vi "GUI_laptop v10.vi"() -> ()   [LabVIEW 2019]
uses:
  <vilib>/Math Plots/3D Math Plots/3D Scatter/3D Scatter XCtrl/3D Scatter.xctl
  <vilib>/Platform/TimedLoop/XDataNode/timing_clust.ctl
  <vilib>/Platform/TimedLoop/XDataNode/nitl_modes.ctl
  <vilib>/Platform/TimedLoop/XDataNode/wakeup.ctl
  <vilib>/Analysis/_algsub.llb/Real Vector Norm.vi
  <vilib>/Instr/_visa.llb/VISA Configure Serial Port (Instr).vi
  <vilib>/Utility/file.llb/Write Delimited Spreadsheet (DBL).vi
  <vilib>/Math Plots/3D Math Plots/3D Scatter/3D Scatter Datatype/Public/Plot Helper (Vector).vi
  <vilib>/platform/TimedLoop/XDataNode/XDataNode.xnode
  <vilib>/Platform/TimedLoop/XDataNode/XDNodeRunTimeDep.lvlib
  <vilib>/Analysis/NI_AALPro.lvlib
  <vilib>/Math Plots/3D Math Plots/3D Scatter/3D Scatter Datatype/3D Scatter Datatype.lvclass
panel:
  out "send values":dbl[](array[numeric])
  out "Robot Feedback (xyz)":dbl[](array[numeric])
  in  "UDP Send":bool
  in  "UDP Recv":bool
  in  "L5 bound":dbl=1000.0
  in  "L4 bound (deg)":dbl=1000.0
  in  "L3 bound (mm)":dbl=1000.0
  in  "L2 bound (deg)":dbl=1000.0
  in  "L1 bound (deg)":dbl=1000.0
  in  "Joystick Type":dbl(ring) items=["Rigid Joystick", "Free Joystick"]
  out "Finished Late? [i-1]":bool
  in  "Epsilon":dbl=0.2
  out "3D Scatter":refnum<class "3D Plot Datatype.lvclass">[](xcontrol)
  out "Random Point":dbl[](array[numeric])
  out "Virtual Cursor":dbl[](array[numeric])
  out "Iteration Duration":i64
  in  "Num of Points":i32=10
  in  "z bound":dbl=2.0
  in  "y bound":dbl=5.0
  in  "x bound":dbl=5.0
  in  "Stop":bool
  in  "Round Decimals":dbl=2.0 format="%#_15g"
  in  "Save  Data":bool
  in  "Save Path":path
  in  "x speed":dbl=0.5
  in  "z speed":dbl=0.5
  in  "y speed":dbl=0.5
  out "error out":errorcluster
  in  "baud rate":u32=115200
  in  "VISA resource name":refnum<visa-resource-name>
  # "TODO: fix the bounds; currently bounds are arbitrary"
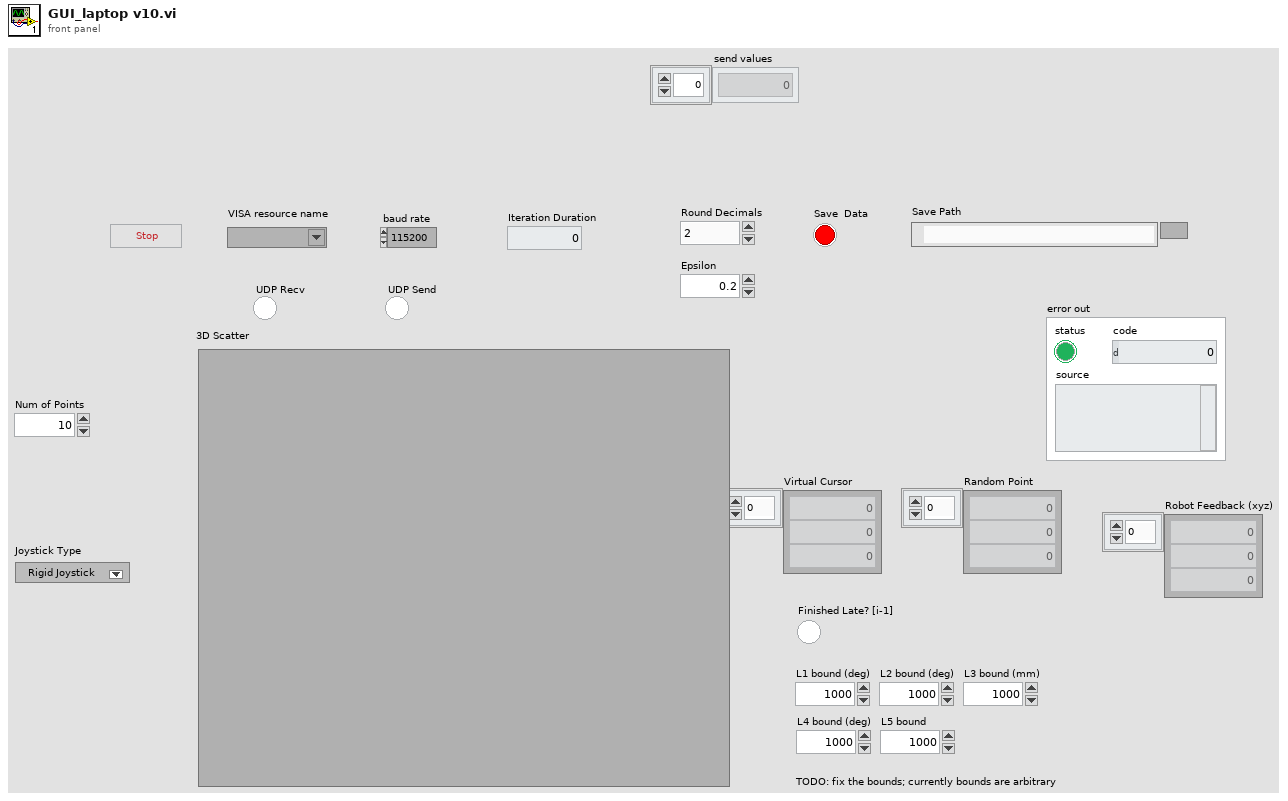
[diagram p1: front panel]
types:
  T1 = typedef "XDNodeRunTimeDep.lvlib/timing_clust.ctl" = cluster{"Expected End [f-1]":u64, "Actual End [f-1]":u64, "Finished Late? [f-1]":bool, "Expected End [i-1]":u64, "Actual End [i-1]":u64, "Finished Late? [i-1]":bool, "Expected Start [i]":u64, "Actual Start [i]":u64, "Expected Start [f]":u64, "Actual Start [f]":u64, "Source Name":string, "Structure Name":string, "Period":i64, "Deadline":i64, "Offset":i64, "Start":i64, "Priority":i32, "Timeout":i32, "Mode":T2, "Wakeup Reason":T3, "Error":errorcluster, "Source Type":string, "Secondary Source Type":string, "Global End Time":u64, "Global Start Time":u64, "Frame Duration":u64, "Iteration Duration":u64, "Assigned CPU":i32, "I/O Scan Engine Mode":u32}
  T2 = typedef "XDNodeRunTimeDep.lvlib/nitl_modes.ctl" = enum32{"No Change", "Process missed periods, maintain original phase", "Discard missed periods, maintain original phase", "Process missed periods, ignore original phase", "Discard missed periods, ignore original phase"}
  T3 = typedef "XDNodeRunTimeDep.lvlib/wakeup.ctl" = enum32{"Normal", "Aborted", "Asynchronous wakeup", "Timing source error", "Timed loop error", "Timeout"}
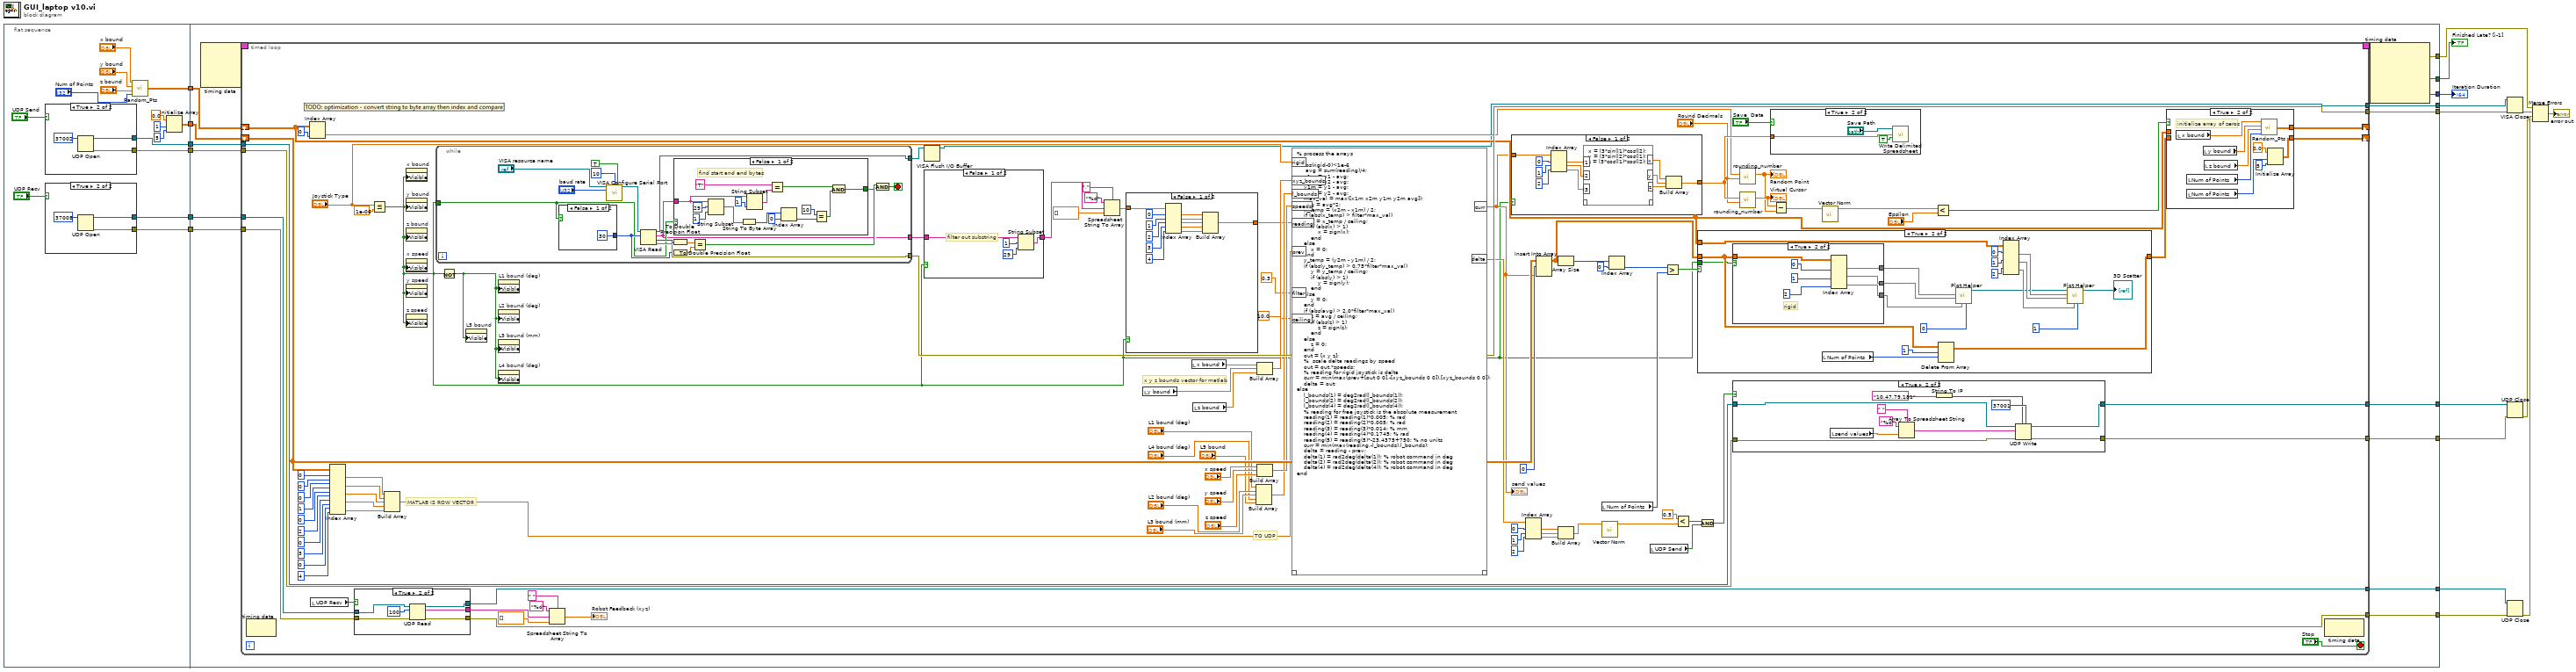
[diagram p0: block diagram]
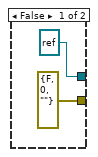
[diagram p2: hidden frame]
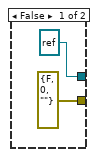
[diagram p3: hidden frame]
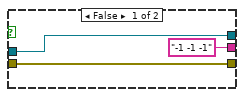
[diagram p5: hidden frame]
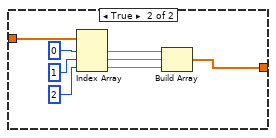
[diagram p9: hidden frame]
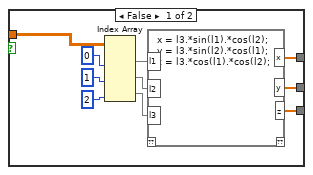
[diagram p12: hidden frame]
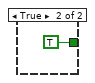
[diagram p13: hidden frame]
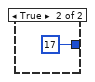
[diagram p14: hidden frame]
diagram:
  n1 = flat-sequence {
    tunnel: [w26] -> w15
    tunnel: [w30] -> w14
    tunnel: [w25] -> w13
    tunnel: [w24] -> w12
    tunnel: [w21] -> w11
    tunnel: [w20] -> w10
    tunnel: [w59] -> w19
    tunnel: [w58] -> w18
    tunnel: [w56] -> w9
    tunnel: [w54] -> w17
    tunnel: [w53] -> w16
    tunnel: w15 -> [w57]
    tunnel: w14 -> [w55]
    tunnel: w13 -> [w52]
    tunnel: w12 -> [w51]
    tunnel: w11 -> [w50]
    tunnel: w10 -> [w49]
    tunnel: [w48] -> w3
    tunnel: [w47] -> w8
    tunnel: [w46] -> w2
    tunnel: [w45] -> w1
    frame #0 {
      n2 = case shown="True" "UDP Send" {
        tunnel: [refnum<k16> refnum ("port") w38] -> w25
        tunnel: [errorcluster {"status"=FALSE, "code"=0, "source"=""} ("error out") w37] -> w20
        frame False {
        }
        frame True {
          n3 = UDP Open(11:u16 37002 ("port")) -> (port=w38:refnum<k16>, 0:w37:errorcluster)  [unwired: 4 in, 1 out]
        }
      }
      n4 = case shown="True" "UDP Recv" {
        tunnel: [refnum<k16> refnum ("port") w43] -> w24
        tunnel: [errorcluster {"status"=FALSE, "code"=0, "source"=""} ("error out") w42] -> w21
        frame False {
        }
        frame True {
          n5 = UDP Open(11:u16 37008 ("port")) -> (port=w43:refnum<k16>, 0:w42:errorcluster)  [unwired: 4 in, 1 out]
        }
      }
      n6 = call "Random_Pts.vi"("Num of Points"="Num of Points", "z bound"="z bound", "y bound"="y bound", "x bound"="x bound") -> ("appended array"=w30:dbl[][])
      n7 = Initialize Array(0.0 ("element"), 1 ("dimension size"), 5 ("dimension size")) -> (w26:dbl[][])
    }
    frame #1 {
      n8 = node-c288() -> (w61:T1)  [unwired: 4 in]
      n9 = timed-loop {
        tunnel: [w94] -> w59
        tunnel: [w158] -> w58
        shift-right: [w157] -> _
        shift-left: w57 -> [w156]
        timing: w61 -> [_]
        timing-out: [_] -> w60
        shift-right: [w152] -> _
        shift-left: w55 -> [w153]
        tunnel: w52 -> [w93]
        tunnel: w51 -> [w92]
        tunnel: w50 -> [w90]
        tunnel: w49 -> [w89]
        tunnel: [w88] -> w48
        tunnel: [w87] -> w47
        tunnel: [w86] -> w46
        tunnel: [w85] -> w45
        stop <- "Stop" stop-if-true
        # "TO UDP"
        # "MATLAB IS ROW VECTOR"
        # "x y z bounds vector for matlab"
        n10 = node-c288() -> ()  [unwired: 1 in, 1 out]
        n11 = Index Array(array=w153, index (col)=0 ("index (row)")) -> (element=w105:dbl[])  [unwired: 1 in]
        n12 = local read "UDP Recv"() -> (w91:bool)
        n13 = Index Array(array=w156, index (row) #1=0 ("disabled index (row)"), index (col) #1=0 ("disabled index (col)"), index (row) #2=0 ("disabled index (row)"), index (col) #2=1 ("disabled index (col)"), index (row) #3=0 ("disabled index (row)"), index (col) #3=2 ("disabled index (col)"), index (row) #4=0 ("disabled index (row)"), index (col) #4=3 ("disabled index (col)"), index (row) #5=0 ("disabled index (row)"), index (col) #5=4 ("disabled index (col)")) -> (element #1=w129:dbl, element #2=w128:dbl, element #3=w127:dbl, element #4=w113:dbl, element #5=w112:dbl)
        n14 = case shown="True" w91 {
          tunnel: w92 -> [w174 w181]
          tunnel: w90 -> [w175 w180]
          tunnel: [w175 w179] -> w88
          tunnel: [w174 w178] -> w86
          tunnel: ["-1 -1 -1" w176] -> w81
          frame False {
          }
          frame True {
            n15 = UDP Read(connection ID=w181, max size (548)=100, 8:w180) -> (data out=w176:string, error out=w179:errorcluster, 3:w178:refnum<k16>)  [unwired: 1 in, 2 out]
          }
        }
        n16 = Less Or Equal?(x="Joystick Type", y=1e-06) -> (x <= y?=w65:bool)
        n17 = Build Array(w129, w128, w127, w113, w112) -> (w126:dbl[])
        n18 = property on="x bound" class="DigNum (strict)"("Visible"=w65) -> ()  [unwired: 2 in, 2 out]
        n19 = property on="y bound" class="DigNum (strict)"("Visible"=w65) -> ()  [unwired: 2 in, 2 out]
        n20 = property on="z bound" class="DigNum (strict)"("Visible"=w65) -> ()  [unwired: 2 in, 2 out]
        n21 = property on="x speed" class="DigNum (strict)"("Visible"=w65) -> ()  [unwired: 2 in, 2 out]
        n22 = property on="y speed" class="DigNum (strict)"("Visible"=w65) -> ()  [unwired: 2 in, 2 out]
        n23 = property on="z speed" class="DigNum (strict)"("Visible"=w65) -> ()  [unwired: 2 in, 2 out]
        n24 = while {
          tunnel: [w270] -> w107
          tunnel: [w283] -> w158
          tunnel: [w277] -> w95
          tunnel: w65 -> [w271]
          stop <- w273 stop-if-true
          n25 = case shown="False" w271 {
            tunnel: [30 u32 17 ("byte count")] -> w276
            frame False {
            }
            frame True {
            }
          }
          n26 = call-poly "VISA Configure Serial Port"("VISA resource name"="VISA resource name", "termination char\n(0xA = '\\n' = LF)"=u8 10 ("termination char\n(0xA = '\\n' = LF)"), "Enable Termination\nChar (T)"=TRUE ("Enable Termination\nChar (T)"), "baud rate (9600)"="baud rate") -> ("VISA resource name out"=w278:refnum<visa-resource-name>)  [unwired: 10 in, 1 out]
          n27 = VISA Read(VISA resource name=w278, byte count=w276) -> (VISA resource name out=w277:refnum<visa-resource-name>, read buffer=w270:string, return count=w285:u32, error out=w283:errorcluster)  [unwired: 1 in]
          n28 = To Double Precision Float(number=w285) -> (double precision float=w284:dbl)
          n29 = To Double Precision Float(number=w276) -> (double precision float=w275:dbl)
          n30 = case shown="False" w271 {
            tunnel: [w292 TRUE] -> w272
            tunnel: w270 -> [w295 _]
            frame False {
              # "find start and end bytes"
              n31 = String Subset(string=w295, offset (0)=29, length (rest)=1) -> (substring=w290:string)
              n32 = String To Byte Array(string=w290) -> (unsigned byte array=w289:u8[])
              n33 = String Subset(string=w295, length (rest)=1) -> (substring=w298:string)  [unwired: 1 in]
              n34 = Equal?(x="T", y=w298) -> (x = y?=w294:bool)
              n35 = Index Array(array=w289, index=0) -> (element=w287:u8)
              n36 = Equal?(x=10, y=w287) -> (x = y?=w293:bool)
              n37 = And(x=w294, y=w293) -> (x .and. y?=w292:bool)
            }
            frame True {
            }
          }
          n38 = Equal?(x=w284, y=w275) -> (x = y?=w274:bool)
          n39 = And(x=w274, y=w272) -> (x .and. y?=w273:bool)
        }
        n40 = Not(x=w65) -> (.not. x?=w64:bool)
        n41 = property on="L5 bound" class="DigNum (strict)"("Visible"=w64) -> ()  [unwired: 2 in, 2 out]
        n42 = property on="L1 bound (deg)" class="DigNum (strict)"("Visible"=w64) -> ()  [unwired: 2 in, 2 out]
        n43 = property on="L2 bound (deg)" class="DigNum (strict)"("Visible"=w64) -> ()  [unwired: 2 in, 2 out]
        n44 = property on="L3 bound (mm)" class="DigNum (strict)"("Visible"=w64) -> ()  [unwired: 2 in, 2 out]
        n45 = property on="L4 bound (deg)" class="DigNum (strict)"("Visible"=w64) -> ()  [unwired: 2 in, 2 out]
        n46 = Spreadsheet String To Array(delimiter (Tab)=" ", format string="%d", spreadsheet string=w81, array type (2D Dbl)=dbl[] []) -> (array=→"Robot Feedback (xyz)":dbl[])
        n47 = VISA Flush I/O Buffer(VISA resource name=w95) -> (VISA resource name out=w94:refnum<visa-resource-name>)  [unwired: 2 in, 1 out]
        n48 = case shown="False" w65 {
          tunnel: w107 -> [w199 w200]
          tunnel: [w196 w200] -> w106
          frame False {
            # "filter out substring"
            n49 = String Subset(string=w199, offset (0)=1, length (rest)=29) -> (substring=w196:string)
          }
          frame True {
          }
        }
        n50 = Spreadsheet String To Array(delimiter (Tab)=",", format string="%d", spreadsheet string=w106, array type (2D Dbl)=dbl[] []) -> (array=w109:dbl[])
        n51 = case shown="False" w65 {
          tunnel: w109 -> [w201 w214]
          tunnel: [w206 w213] -> w108
          frame False {
            n52 = Index Array(array=w201, index #1=0 ("Plot ID"), index #2=1 ("Plot ID"), index #3=2 ("Plot ID"), index #4=3 ("Plot ID"), index #5=4 ("Plot ID")) -> (element #1=w209:dbl, element #2=w208:dbl, element #3=w207:dbl, element #4=w203:dbl, element #5=w202:dbl)
            n53 = Build Array(w209, w208, w207, w203, w202) -> (w206:dbl[])
          }
          frame True {
            n54 = Index Array(array=w214, index #1=0 ("Plot ID"), index #2=1 ("Plot ID"), index #3=2 ("Plot ID")) -> (element #1=w217:dbl, element #2=w216:dbl, element #3=w215:dbl)
            n55 = Build Array(w217, w216, w215) -> (w213:dbl[])
          }
        }
        n56 = local read "y bound"() -> (w131:dbl)
        n57 = local read "x bound"() -> (w132:dbl)
        n58 = local read "z bound"() -> (w130:dbl)
        n59 = Build Array("L1 bound (deg)", "L2 bound (deg)", "L3 bound (mm)", "L4 bound (deg)", "L5 bound") -> (w120:dbl[])
        n60 = Build Array(w132, w131, w130) -> (w124:dbl[])
        n61 = Build Array("x speed", "y speed", "z speed") -> (w125:dbl[])
        n62 = script code="% process the arrays\n\nif abs(rigid-0)<1e-6\n     avg = sum(reading)/4;\n    x1m = x1 - avg;\n    x2m = x2 - avg;\n    y1m = y1 - avg;\n    y2m = y2 - avg;\n    max_val = max([x1m x2m y1m y2m avg]);\n    avg = avg*2;\n    x_temp = (x2m - x1m) / 2;\n    if (abs(x_temp) > filter*max_val)\n        x = x_temp / ceiling;\n        if (abs(x) > 1)\n            x = sign(x);\n        end\n    else\n        x = 0;\n    end\n    y_temp = (y2m - y1m) / 2;\n    if (abs(y_temp) > 0.75*filter*max_val)\n        y = y_temp / ceiling;\n        if (abs(y) > 1)\n            y = sign(y);\n        end\n    else\n        y = 0;\n    end\n    if (abs(avg) > 2.0*filter*max_val)\n        z = avg / ceiling;\n        if (abs(z) > 1)\n            z = sign(z);\n        end\n    else\n        z = 0;\n    end\n    out = [x y z];\n    %  scale delta readings by speed\n    out = out.*speeds;\n    % reading for rigid joystick is delta\n    curr = min(max(prev+[out 0 0],-[xyz_bounds 0 0]),[xyz_bounds 0 0]);\n    delta = out;\nelse\n    l_bounds(1) = deg2rad(l_bounds(1));\n    l_bounds(2) = deg2rad(l_bounds(2));\n    l_bounds(4) = deg2rad(l_bounds(4));\n    % reading for free joystick is the absolute measurement\n    reading(1) = reading(1)*0.005; % rad\n    reading(2) = reading(2)*0.005; % rad\n    reading(3) = reading(3)*0.014; % mm\n    reading(4) = reading(4)*0.1745; % rad\n    reading(5) = reading(5)*-23.4375+750; % no units\n    curr = min(max(reading,-l_bounds),l_bounds);\n    delta = reading - prev;\n    delta(1) = rad2deg(delta(1)); % robot command in deg\n    delta(2) = rad2deg(delta(2)); % robot command in deg\n    delta(4) = rad2deg(delta(4)); % robot command in deg\nend"("xyz_bounds"=w124, "speeds"=w125, "reading"=w108, "prev"=w126, "rigid"="Joystick Type", "l_bounds"=w120, "filter"=0.3 ("Real"), "ceiling"=10.0 ("Real")) -> ("curr"=w66:dbl[], "delta"=w74:dbl[])  [unwired: 1 in, 1 out]
        "send values" <- w66
        n63 = case shown="False" w65 {
          tunnel: w66 -> [w228 w232]
          tunnel: [w221 w232] -> w154
          frame False {
            n64 = Index Array(array=w228, index #1=0 ("Plot ID"), index #2=1 ("Plot ID"), index #3=2 ("Plot ID")) -> (element #1=w227:dbl, element #2=w226:dbl, element #3=w225:dbl)
            n65 = script code="x = l3*sin(l1)*cos(l2);\ny = l3*sin(l2)*cos(l1);\nz = l3*cos(l1)*cos(l2);"("l1"=w227, "l2"=w226, "l3"=w225) -> ("x"=w224:dbl, "y"=w223:dbl, "z"=w222:dbl)  [unwired: 1 in, 1 out]
            n66 = Build Array(w224, w223, w222) -> (w221:dbl[])
          }
          frame True {
          }
        }
        n67 = Index Array(array=w74, index #1=0 ("disabled index (col)"), index #2=1 ("disabled index (col)"), index #3=2 ("disabled index (col)")) -> (element #1=w70:dbl, element #2=w69:dbl, element #3=w68:dbl)
        n68 = Insert Into Array(array=w156, index (row)=0, new element=w66) -> (w137:dbl[][])  [unwired: 1 in]
        n69 = Array Size(array=w137) -> (size(s)=w139:i32[])
        n70 = Build Array(w70, w69, w68) -> (w67:dbl[])
        n71 = local read "Num of Points"() -> (w138:i32)
        n72 = call-poly <vilib>:"Vector Norm.vi"("Input Vector"=w67) -> ("norm"=w79:dbl)  [unwired: 9 in, 1 out]
        n73 = Index Array(array=w139, index=0) -> (element=w140:i32)
        n74 = local read "UDP Send"() -> (w76:bool)
        n75 = Greater?(x=w140, y=w138) -> (0:w136:bool)
        n76 = Less?(x=0.5, y=w79) -> (x < y?=w77:bool)
        n77 = case shown="True" w136 {
          tunnel: w137 -> [w233 w251]
          tunnel: [w233 w250] -> w155
          tunnel: w153 -> [_ w249]
          tunnel: w65 -> [_ w234]
          frame False {
          }
          frame True {
            n78 = case shown="True" w234 {
              tunnel: w251 -> [w262 w266]
              tunnel: [w253 w265] -> w240
              tunnel: [w254 w264] -> w239
              tunnel: [w255 w263] -> w238
              frame False {
                n79 = Index Array(array=w262, index (col) #1=0 ("Plot ID"), index (col) #2=1 ("Plot ID"), index (col) #3=2 ("Plot ID")) -> (element #1=w258:dbl[], element #2=w257:dbl[], element #3=w256:dbl[])  [unwired: 3 in]
                n80 = script code="x = l3.*sin(l1).*cos(l2);\ny = l3.*sin(l2).*cos(l1);\nz = l3.*cos(l1).*cos(l2);"("l1"=w258, "l2"=w257, "l3"=w256) -> ("x"=w253:dbl[], "y"=w254:dbl[], "z"=w255:dbl[])  [unwired: 1 in, 1 out]
              }
              frame True {
                # "rigid"
                n81 = Index Array(array=w266, index (col) #1=0 ("disabled index (col)"), index (col) #2=1 ("index (col)"), index (col) #3=2 ("index (col)")) -> (element #1=w265:dbl[], element #2=w264:dbl[], element #3=w263:dbl[])  [unwired: 3 in]
              }
            }
            n82 = local read "Num of Points"() -> (w248:i32)
            n83 = Delete From Array(array=w251, length=1, index (row)=w248) -> (array with subset deleted=w250:dbl[][])  [unwired: 1 in, 1 out]
            n84 = call-poly <vilib>:"Plot Helper.vi"("Plot ID"=0, "z vector"=w238, "y vector"=w239, "x vector"=w240) -> ("3D Plot lvclass Array out"=w242:refnum<class "3D Plot Datatype.lvclass">[])  [unwired: 2 in, 5 out]
            n85 = Index Array(array=w249, index (row) #1=0 ("index (row)"), index (row) #2=1 ("index (row)"), index (row) #3=2 ("index (row)")) -> (element #1=w246:dbl[], element #2=w245:dbl[], element #3=w244:dbl[])  [unwired: 3 in]
            n86 = call-poly <vilib>:"Plot Helper.vi"("Plot ID"=1, "z vector"=w244, "y vector"=w245, "x vector"=w246, "3D Plot lvclass Array in"=w242) -> ("3D Plot lvclass Array out"=→"3D Scatter":refnum<class "3D Plot Datatype.lvclass">[])  [unwired: 1 in, 5 out]
          }
        }
        n87 = And(x=w77, y=w76) -> (x .and. y?=w75:bool)
        n88 = case shown="True" w75 {
          tunnel: w93 -> [w160 w172]
          tunnel: w89 -> [w161 w168]
          tunnel: [w161 w164] -> w87
          tunnel: [w160 w163] -> w85
          frame False {
          }
          frame True {
            n89 = local read "send values"() -> (w162:dbl[])
            n90 = Array To Spreadsheet String(delimiter (Tab)=" ", array=w162, 3:"%d" ("format string")) -> (spreadsheet string=w169:string)
            n91 = String To IP(1:"10.47.79.181" ("name")) -> (0:w166:u32)
            n92 = UDP Write(address=w166, port or service name=u16 37001, connection ID=w172, data in=w169, 8:w168) -> (error out=w164:errorcluster, 3:w163:refnum<k16>)  [unwired: 1 in]
          }
        }
        n93 = call "rounding_number.vi"("power of ten"="Round Decimals", "Array"=w105) -> ("rounded"=w101:dbl[])  [unwired: 9 in]
        "Random Point" <- w101
        n94 = call "rounding_number.vi"("power of ten"="Round Decimals", "Array"=w154) -> ("rounded"=w102:dbl[])  [unwired: 9 in]
        "Virtual Cursor" <- w102
        n95 = case shown="True" "Save  Data" {
          tunnel: w154 -> [_ w182]
          frame False {
          }
          frame True {
            n96 = call-poly <vilib>:"Write Delimited Spreadsheet.vi"("file path (dialog if empty)"="Save Path", "1D data"=w182, "append to file? (new file:F)"=TRUE) -> ()  [unwired: 11 in, 2 out]
          }
        }
        n97 = Subtract(x=w102, y=w101) -> (x-y=w100:dbl[])
        n98 = call-poly <vilib>:"Vector Norm.vi"("Input Vector"=w100) -> ("norm"=w99:dbl)  [unwired: 9 in, 1 out]
        n99 = Less?(x=w99, y="Epsilon") -> (x < y?=w97:bool)
        n100 = case shown="True" w97 {
          tunnel: w153 -> [w186 _]
          tunnel: [w186 w191] -> w152
          tunnel: w155 -> [w185 _]
          tunnel: [w185 w187] -> w157
          frame False {
          }
          frame True {
            # "initialize array of zeros"
            n101 = local read "x bound"() -> (w195:dbl)
            n102 = local read "Num of Points"() -> (w192:i32)
            n103 = local read "Num of Points"() -> (w189:i32)
            n104 = local read "y bound"() -> (w194:dbl)
            n105 = local read "z bound"() -> (w193:dbl)
            n106 = call "Random_Pts.vi"("Num of Points"=w192, "z bound"=w193, "y bound"=w194, "x bound"=w195) -> ("appended array"=w191:dbl[][])
            n107 = Initialize Array(0.0 ("element"), w189, 5 ("dimension size")) -> (w187:dbl[][])
          }
        }
        n108 = node-c288() -> ()  [unwired: 1 in, 1 out]
      }
      n109 = node-c288(w60) -> (w56:errorcluster, w53:bool, w54:i64)  [unwired: 3 out]
    }
  }
  n110 = VISA Close(VISA resource name=w19, error in (no error)=w18) -> (error out=w7:errorcluster)
  n111 = UDP Close(connection ID=w1, 8:w8) -> (error out=w5:errorcluster)  [unwired: 1 out]
  n112 = UDP Close(connection ID=w2, 8:w3) -> (error out=w6:errorcluster)  [unwired: 1 out]
  n113 = Merge Errors(w9, w7, w6, w5) -> (→"error out":errorcluster)
  "Iteration Duration" <- w17
  "Finished Late? [i-1]" <- w16
